vi "DataLog Format Point Value.vi"(7 "value":dbl format="%.17e", 11 "tag config":T1 {"logging parameters" format="%.2e"; "precision" items=["0", "1", "2", "3", "4", "5", "6", "7", "8", "9", "10", "11", "12", "13", "14", "15", "16", "17"]; "limit delay" format="%.2e"; "deadband" format="%.2e"}) -> (8 "formatted value":string)   [LabVIEW 2012]
doc: "This VI formats a tag's point value to a string as per the formatting specifiers and value type found in tag's configuration."
uses:
  typedefs/clusters/t_DataLog Tag Config.ctl
  typedefs/t_DataLog Temporal Types.ctl
  typedefs/t_DataLog Value Types.ctl
  typedefs/t_DataLog Numerical Format.ctl
  typedefs/t_DataLog Logging Algorithms.ctl
  glb_DataLog MCVD.vi
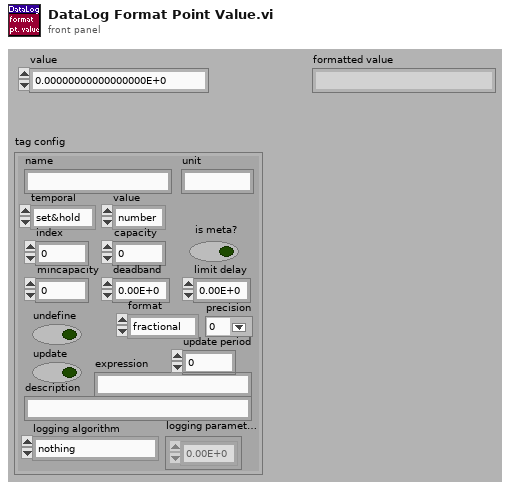
[diagram p1: front panel]
types:
  T1 = typedef "t_DataLog Tag Config.ctl" = cluster{"name":string, "unit":string, "temporal":T2, "value":T3, "index":i32, "capacity":i32, "is meta?":bool, "mincapacity":i32, "deadband":dbl, "limit delay":dbl, "format":T4, "precision":u8, "undefine":bool, "update":bool, "update period":u16, "expression":string, "description":string, "logging algorithm":T5, "logging parameters":dbl[]}
  T2 = typedef "t_DataLog Temporal Types.ctl" = enum16{"set&hold", "sample", "event"}
  T3 = typedef "t_DataLog Value Types.ctl" = enum16{"number", "string"}
  T4 = typedef "t_DataLog Numerical Format.ctl" = enum8{"fractional", "exponential", "engineering"}
  T5 = typedef "t_DataLog Logging Algorithms.ctl" = enum16{"nothing", "changes", "everything", "every Nth", "time threshold", "value threshold + prior", "t or v threshold", "t or v threshold + prior"}
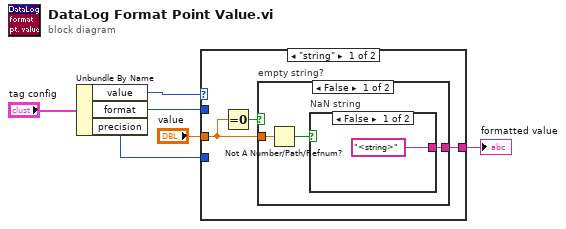
[diagram p0: block diagram]
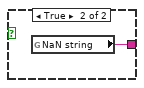
[diagram p2: hidden frame]
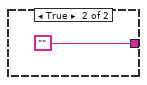
[diagram p3: hidden frame]
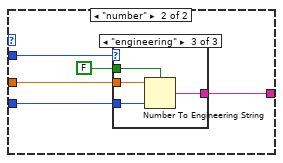
[diagram p4: hidden frame]
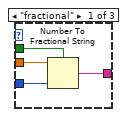
[diagram p5: hidden frame]
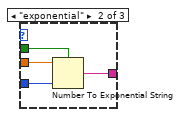
[diagram p6: hidden frame]
diagram:
  n1 = Unbundle By Name("tag config") -> ("value"=w1:T3, "format"=w3:T4, "precision"=w2:u8)
  n2 = case shown="\"string\"" w1 {
    tunnel: "value" -> [w7 w20]
    tunnel: [w8 w19] -> w5
    tunnel: w3 -> [_ w17]
    tunnel: w2 -> [_ w16]
    frame "string" {
      n3 = Equal To 0?(x=w7) -> (x = 0?=w9:bool)
      n4 = case "empty string?" shown="False" w9 {
        tunnel: [w10 ""] -> w8
        tunnel: w7 -> [w12 _]
        frame False {
          n5 = Not A Number/Path/Refnum?(number/path/refnum=w12) -> (NaN/Path/Refnum?=w11:bool)
          n6 = case "NaN string" shown="False" w11 {
            tunnel: ["<string>" ("NaN string") w14] -> w10
            frame False {
            }
            frame True {
              n7 = global read "glb_DataLog MCVD.vi" "NaN string"() -> (w14:string)
            }
          }
        }
        frame True {
        }
      }
    }
    frame "number" {
      n8 = case shown="\"engineering\"" w17 {
        tunnel: w20 -> [w24 w28 w32]
        tunnel: w16 -> [w23 w27 w31]
        tunnel: [w22 w26 w30] -> w19
        tunnel: FALSE ("use system decimal point (T)") -> [w21 w25 w29]
        frame "fractional" {
          n9 = Number To Fractional String(use system decimal point (T)=w21, number=w24, precision (6)=w23) -> (F-format string=w22:string)  [unwired: 1 in]
        }
        frame "exponential" {
          n10 = Number To Exponential String(number=w28, precision (6)=w27, 1:w25) -> (E-format string=w26:string)  [unwired: 1 in]
        }
        frame "engineering" {
          n11 = Number To Engineering String(1:w29, 2:w31, 4:w32) -> (0:w30:string)  [unwired: 1 in]
        }
      }
    }
  }
  "formatted value" <- w5
